vi "Advanced DC-RMS Measurement Example.vi"() -> (3 "Test Signal":waveform(dbl))   [LabVIEW 2017, in "Examples.lvlib"]
uses:
  Examples.lvlib
  <vilib>/Analysis/NI_AALBase.lvlib
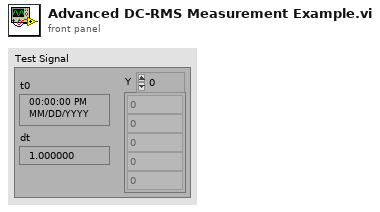
[diagram p1: front panel]
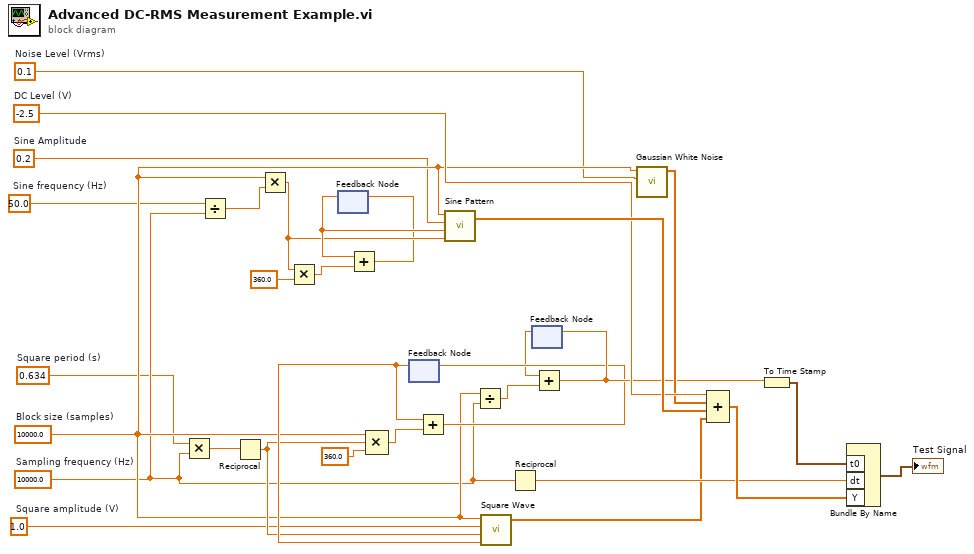
[diagram p0: block diagram]
diagram:
  w4 = 1.0  # Square amplitude (V)
  w15 = 10000.0  # Sampling frequency (Hz)
  w16 = 10000.0  # Block size (samples)
  w9 = 0.634  # Square period (s)
  w1 = 50.0  # Sine frequency (Hz)
  w10 = 0.2  # Sine Amplitude
  w22 = -2.5  # DC Level (V)
  w2 = 0.1  # Noise Level (Vrms)
  n1 = Multiply(x=w9, y=w15) -> (x*y=w8:dbl)
  n2 = Divide(x=w1, y=w15) -> (x/y=w3:dbl)
  n3 = Reciprocal(x=w8) -> (1/x=w23:dbl)
  n4 = Multiply(x=w16, y=w3) -> (x*y=w11:dbl)
  n5 = Multiply(x=w11, y=360.0) -> (x*y=w6:dbl)
  n6 = feedback #1() -> (w12:dbl)  [unwired: 1 in]
  n7 = Add(x=w12, y=w6) -> (x+y=w7:dbl)
  n8 = feedback-in #1(w7) -> ()
  n9 = Compound Arithmetic op=MULTIPLY(w16, w23, 360.0 ("value")) -> (w13:dbl)
  n10 = feedback #2() -> (w24:dbl)  [unwired: 1 in]
  n11 = Add(x=w24, y=w13) -> (x+y=w19:dbl)
  n12 = feedback-in #2(w19) -> ()
  n13 = call <vilib>:"Sine Pattern.vi"("cycles"=w11, "phase(degrees)"=w12, "amplitude"=w10, "samples"=w16) -> ("Sinusoidal Pattern"=w25:dbl[])  [unwired: 1 out]
  n14 = Divide(x=w16, y=w15) -> (x/y=w17:dbl)
  n15 = call <vilib>:"Square Wave.vi"("samples"=w16, "amplitude"=w4, "frequency"=w23, "phase in"=w24) -> ("square wave"=w26:dbl[])  [unwired: 2 in, 2 out]
  n16 = Reciprocal(x=w15) -> (1/x=w28:dbl)
  n17 = feedback #3() -> (w18:dbl)  [unwired: 1 in]
  n18 = Add(x=w18, y=w17) -> (x+y=w20:dbl)
  n19 = feedback-in #3(w20) -> ()
  n20 = call <vilib>:"Gaussian White Noise.vi"("standard deviation"=w2, "samples"=w16) -> ("Gaussian noise pattern"=w21:dbl[])  [unwired: 8 in, 1 out]
  n21 = Compound Arithmetic op=ADD(w22, w21, w25, w26) -> (w29:dbl[])
  n22 = To Time Stamp(1:w20) -> (0:w27:timestamp)
  n23 = Bundle By Name("t0"=w27, "dt"=w28, "Y"=w29) -> (→"Test Signal":waveform(dbl))  [unwired: 1 in]
